vi "Launch Start Actors.vi"(8 "error in (no error)":errorcluster, 11 "CS++StartActor in":refnum<class "CS++StartActor.lvclass">) -> (0 "error out":errorcluster, 3 "CS++StartActor out":refnum<class "CS++StartActor.lvclass">)   [LabVIEW 2012, in "CS++StartActor.lvlib" / "CS++StartActor.lvclass"]
doc: "Launch Start Actors."
uses:
  CS++StartActor.lvclass
  <vilib>/ActorFramework/Actor/Actor.lvclass/Actor.ctl
  <vilib>/ActorFramework/Message Enqueuer/Message Enqueuer.lvclass/Message Enqueuer.ctl
  CS++BaseActor/CS++BaseActor.lvclass/CS++BaseActor.ctl
  CS++StartActor.lvclass/CS++StartActor.ctl
  CS++BaseActor Messages/Open Actor Core FP Msg/Open Actor Core FP Msg.lvclass/Open Actor Core FP Msg.ctl
  <vilib>/ActorFramework/Message Enqueuer/Init from Existing Queue.vi
  <vilib>/ActorFramework/Message Enqueuer/Enqueue.vi
  <vilib>/ActorFramework/Message Priority Queue/Priority Enqueue.vi
  <vilib>/ActorFramework/Message Enqueuer/Message Enqueuer.lvclass
  CS++BaseActor Messages/Open Actor Core FP Msg/Open Actor Core FP Msg.lvclass
  <vilib>/ActorFramework/Actor/Actor.lvclass
  Classes/CS++BaseClasses/Factory/CS++Factory.lvclass
  CS++BaseActor/CS++BaseActor.lvclass
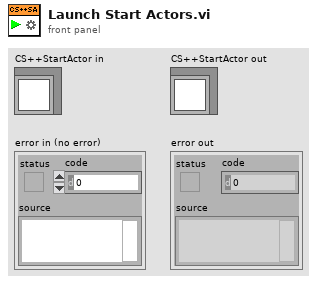
[diagram p1: front panel]
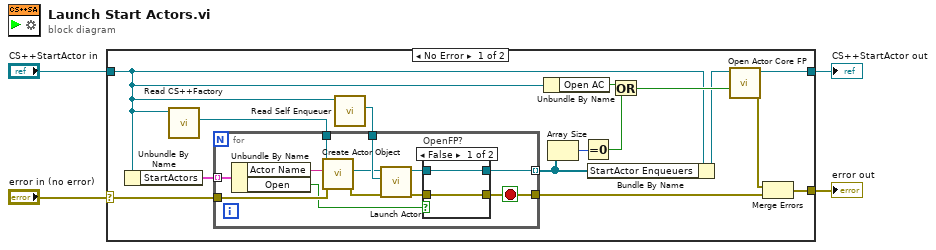
[diagram p0: block diagram]
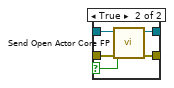
[diagram p2: hidden frame]
diagram:
  n1 = case shown="No Error" "error in (no error)" {
    selector: "error in (no error)" -> [w17 w40]
    tunnel: [w6 w40] -> w3
    tunnel: [w7 w39] -> w1
    tunnel: "CS++StartActor in" -> [w9 w39]
    frame No Error {
      n2 = Unbundle By Name(w9) -> ("StartActors"=w18:cluster{"Actor Name":string, "Open":bool}[])
      n3 = call "Read CS++Factory.vi"("CS++BaseActor in"=w9) -> ("CS++Factory"=w15:refnum<class "CS++Factory.lvclass">)  [unwired: 8 in, 2 out]
      n4 = call <vilib>:"Read Self Enqueuer.vi"("Actor"=w9) -> ("Self Enqueuer"=w19:refnum<class "Message Enqueuer.lvclass">)  [unwired: 10 in]
      n5 = for {
        tunnel: w19 -> [w31]
        tunnel: w18 -> [w26] mode=indexing
        tunnel: w15 -> [w29]
        tunnel: w17 -> [w28]
        tunnel: [w23] -> w16
        tunnel: [w21] -> w14 mode=indexing
        stop <- w23 stop-if-true
        n6 = Unbundle By Name(w26) -> ("Actor Name"=w25:string, "Open"=w20:bool)
        n7 = call "Create Actor Object.vi"("error in (no error)"=w28, "Object Name"=w25, "CS++Factory in"=w29) -> ("error out"=w27:errorcluster, "C++BaseActor"=w30:refnum<class "CS++BaseActor.lvclass">)  [unwired: 5 in, 2 out]
        n8 = call <vilib>:"Launch Actor.vi"("error in (no error)"=w27, "Actor-to-Caller Enqueuer"=w31, "Actor"=w30) -> ("error out"=w24:errorcluster, "Caller-To-Actor Enqueuer"=w22:refnum<class "Message Enqueuer.lvclass">)  [unwired: 7 in]
        n9 = case "OpenFP?" shown="False" w20 {
          selector: w20 -> [_ w34]
          tunnel: w24 -> [w32 w38]
          tunnel: [w32 w37] -> w23
          tunnel: w22 -> [w33 w36]
          tunnel: [w33 w35] -> w21
          frame False {
          }
          frame True {
            n10 = call "Send Open Actor Core FP.vi"("error in (no error)"=w38, "Open FP (F)"=w34, "Message Enqueuer"=w36) -> ("error out"=w37:errorcluster, "Message Enqueuer out"=w35:refnum<class "Message Enqueuer.lvclass">)  [unwired: 7 in]
          }
        }
      }
      n11 = Unbundle By Name(w9) -> ("Open AC"=w11:bool)
      n12 = Array Size(array=w14) -> (size(s)=w13:i32)
      n13 = Equal To 0?(x=w13) -> (x = 0?=w12:bool)
      n14 = Bundle By Name(cluster=w9, "StartActor Enqueuers"=w14) -> (w8:refnum<class "CS++StartActor.lvclass">)
      n15 = Or(x=w11, y=w12) -> (x .or. y?=w10:bool)
      n16 = call "Open Actor Core FP.vi"("Open FP (F)"=w10, "CS++BaseActor in"=w8) -> ("error out"=w5:errorcluster, "CS++BaseActor out"=w7:refnum<class "CS++StartActor.lvclass">)  [unwired: 8 in]
      n17 = Merge Errors(w5, w16) -> (w6:errorcluster)
    }
    frame Error {
    }
  }
  "error out" <- w3
  "CS++StartActor out" <- w1
